vi "Main_07A.vi"() -> ()   [LabVIEW 2025]
uses:
  Utility/Universal Utility/TypeDefs_Utility/Cluster_Row-Column.ctl
  9e3f57c0-2ef8-4495-8287-c6a42a5fb955.vi
  Utility/Universal Utility/TypeDefs_Utility/ENUM_4 Directions U-D-L-R.ctl
  Utility/Universal Utility/TypeDefs_Utility/ENUM_8 Directions U-D-L-R.ctl
  299cb445-af19-43c4-83da-fdf18fff65e6.vi
panel:
  out "MATCH":bool
  in  "Select Data":enum32{"Example", "Puzzle"}(tab)
  in  "EX Target":u64
  in  "Example":string
  in  "Puzzle":string
  in  "Puzzle Target":u64
  out "Answer":u64
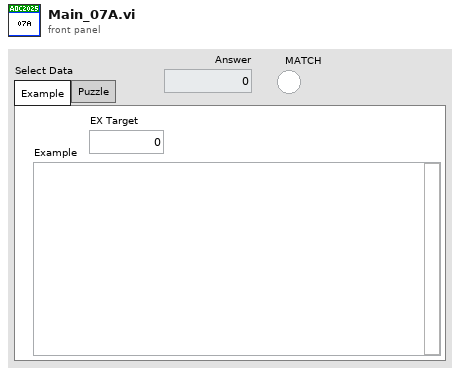
[diagram p1: front panel]
types:
  T1 = typedef "ENUM_4 Directions U-D-L-R.ctl" = enum16{"Up;-1,0", "Right;0,1", "Down;1,0", "Left;0,-1"}
  T2 = typedef "ENUM_8 Directions U-D-L-R.ctl" = enum16{"Up;-1,0", "Up-Right;-1,1", "Right;0,1", "Down-Right;1,1", "Down;1,0", "Down-Left;1,-1", "Left;0,-1", "Up-Left;-1,-1"}
  T3 = typedef "Cluster_Row-Column.ctl" = cluster{"R":i32, "C":i32}
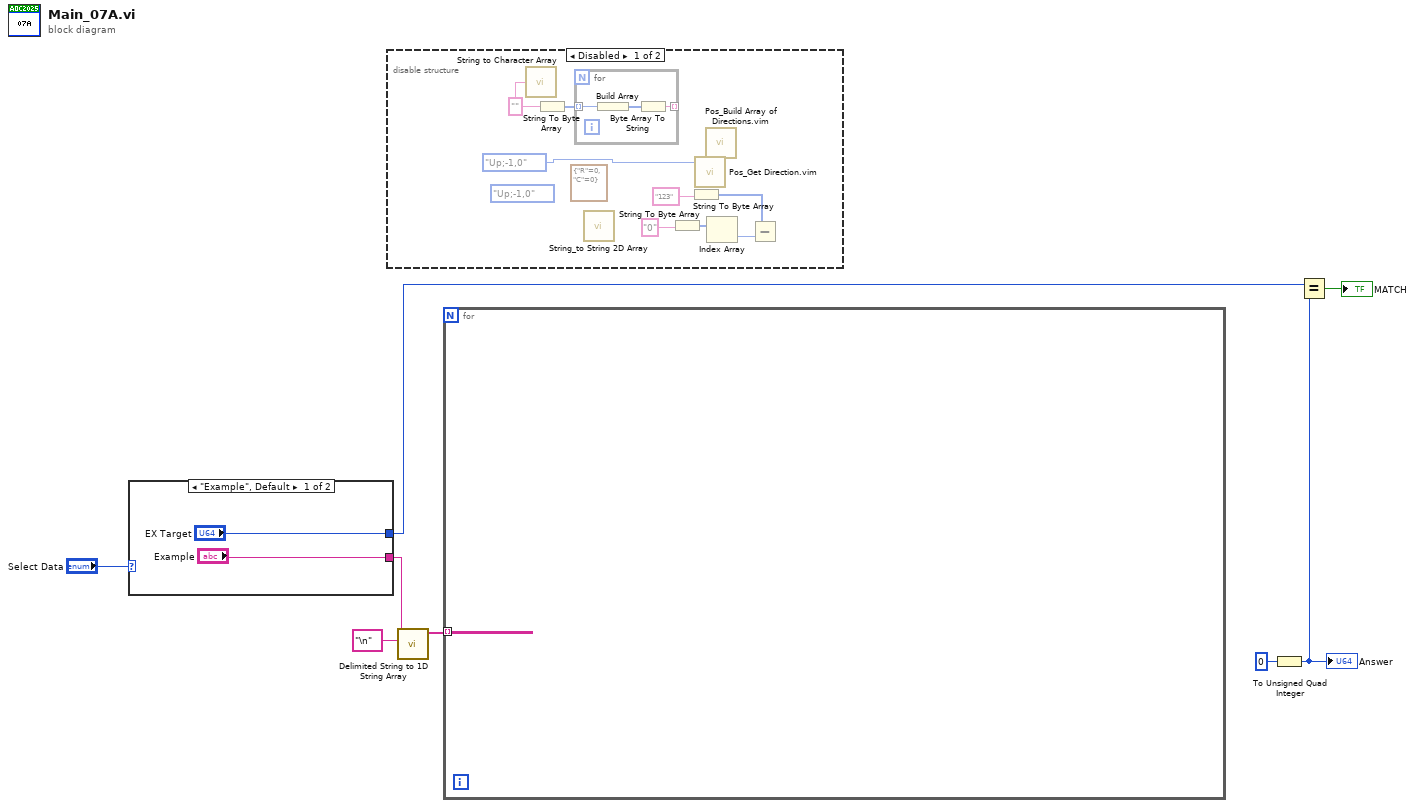
[diagram p0: block diagram]
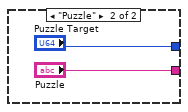
[diagram p2: hidden frame]
diagram:
  n1 = case shown="\"Example\", Default" "Select Data" {
    tunnel: ["Example" "Puzzle"] -> w6
    tunnel: ["EX Target" "Puzzle Target"] -> w3
    frame "Example", Default {
    }
    frame "Puzzle" {
    }
  }
  n2 = disable-structure shown="Disabled" {
    frame Disabled {
      w16 = "" ("string")
      (unwired) ENUM_8_Directions_U-D-L-R."Up;-1,0" ("Direction 8")
      (unwired) T3 {"R"=0, "C"=0} ("Position")
      n3 = call "String to Character Array.vi"("Input String"=w16) -> ()  [unwired: 1 out]
      n4 = String To Byte Array(string=w16) -> (unsigned byte array=w17:u8[])
      n5 = for {
        tunnel: w17 -> [w23] mode=indexing
        tunnel: [w21] -> _ mode=indexing
        n6 = Build Array(w23) -> (w22:u8[])
        n7 = Byte Array To String(unsigned byte array=w22) -> (string=w21:string)
      }
      n8 = call "String_to String 2D Array.vi"() -> ()  [unwired: 11 in, 1 out]
      n9 = String To Byte Array(string="0") -> (unsigned byte array=w20:u8[])
      n10 = String To Byte Array(string="123") -> (unsigned byte array=w18:u8[])
      n11 = call "Pos_Get Direction.vim"("Direction 8"=ENUM_4_Directions_U-D-L-R."Up;-1,0" ("Direction")) -> ()  [unwired: 10 in, 1 out]
      n12 = call "Pos_Build Array of Directions.vim"() -> ()  [unwired: 10 in, 2 out]
      n13 = Index Array(array=w20) -> (element=w19:u8)  [unwired: 1 in]
      n14 = Subtract(x=w18, y=w19) -> ()  [unwired: 1 out]
    }
    frame Enabled {
    }
  }
  n15 = call <vilib>:"Delimited String to 1D String Array.vi"("delimiter"="\n" ("delimiter (Tab)"), "delimited string"=w6) -> ("string array"=w7:string[])  [unwired: 9 in]
  n16 = for {
    tunnel: w7 -> [_] mode=indexing
  }
  n17 = To Unsigned Quad Integer(1:u64 0 ("number")) -> (0:w1:u64)
  "Answer" <- w1
  n18 = Equal?(x=w3, y=w1) -> (x = y?=→"MATCH":bool)
